vi "niRFSysCalReader Optimized Interpolation Method.vi"(0 "Max Delta Frequency, Hz":dbl=inf step=1000000.0 format="%^.6e", 1 "Max Delta Power Level, dBm":dbl=inf step=10.0 format="%.1f", 2 "Table (frequency, power, pathloss)":dbl[][](array[numeric]) caption="Calibration Table [Hz, dBm, dB]" min=0.0 max=127.0 format="%.2p", 3 "Max Input Power, dBm":dbl format="%.1f", 4 "Center Frequency, Hz":dbl=1000000000.0 step=1000000.0 format="%^.6e") -> (5 "Max Frequency Delta Reached?":bool, 6 "Max Power Delta Reached?":bool, 7 "External Attenuation, dB":dbl format="%.2f")   [LabVIEW 2016, in "niRFSysCalReader.lvlib"]
uses:
  niRFSysCalReader.lvlib
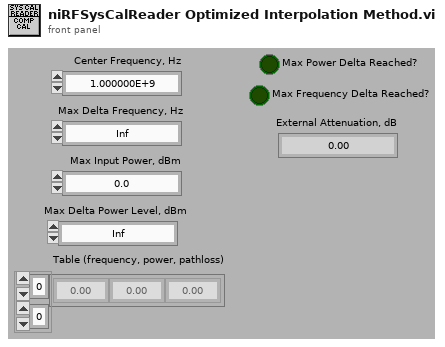
[diagram p1: front panel]
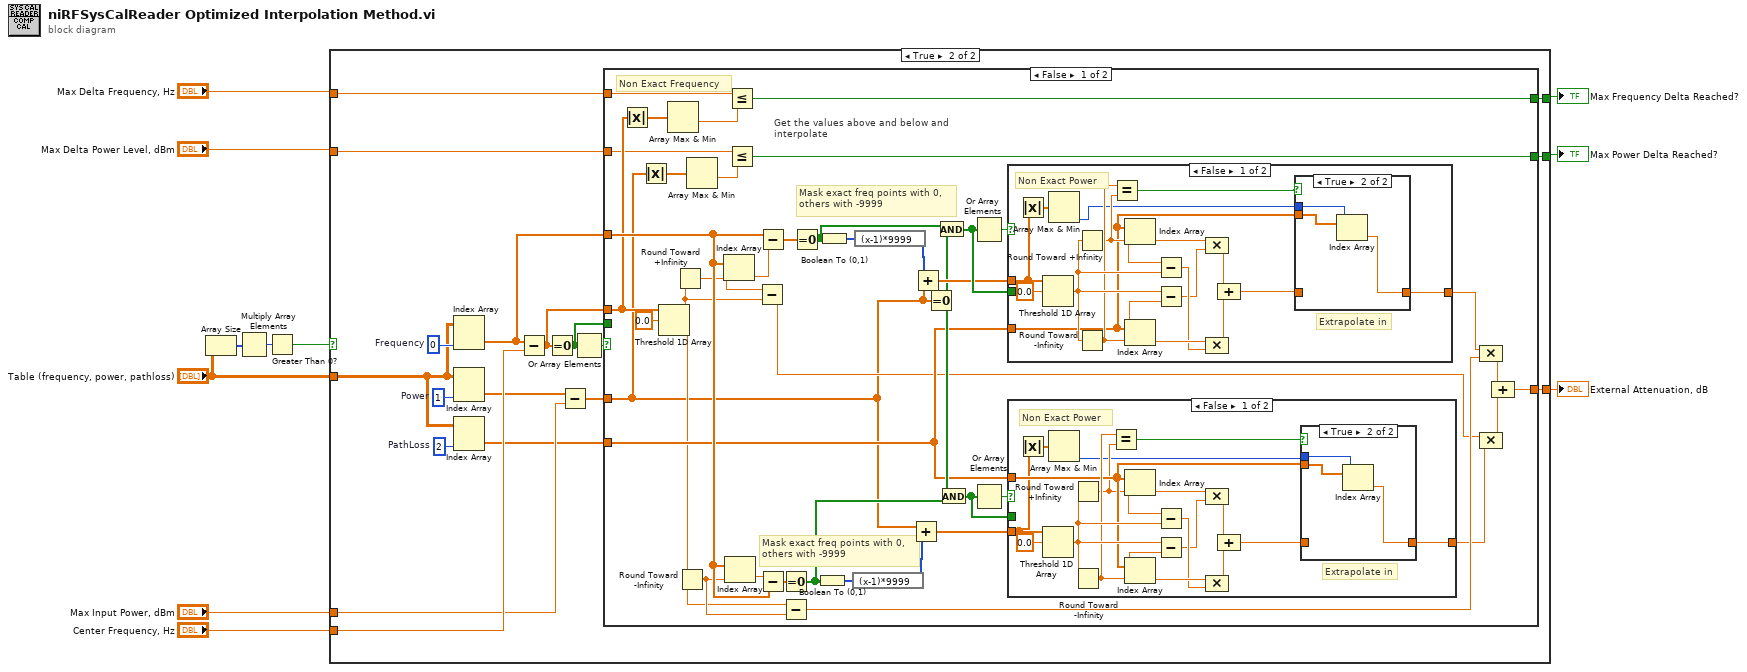
[diagram p0: block diagram]
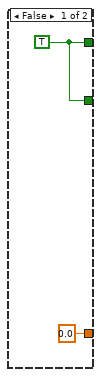
[diagram p2: hidden frame]
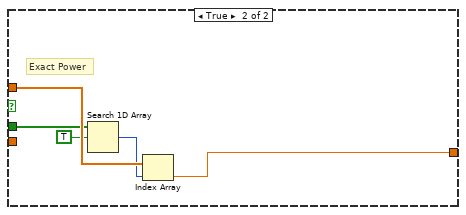
[diagram p4: hidden frame]
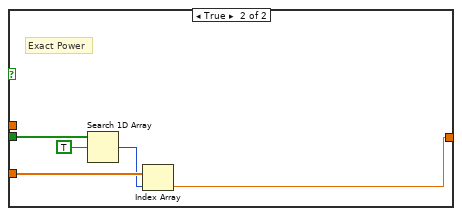
[diagram p6: hidden frame]
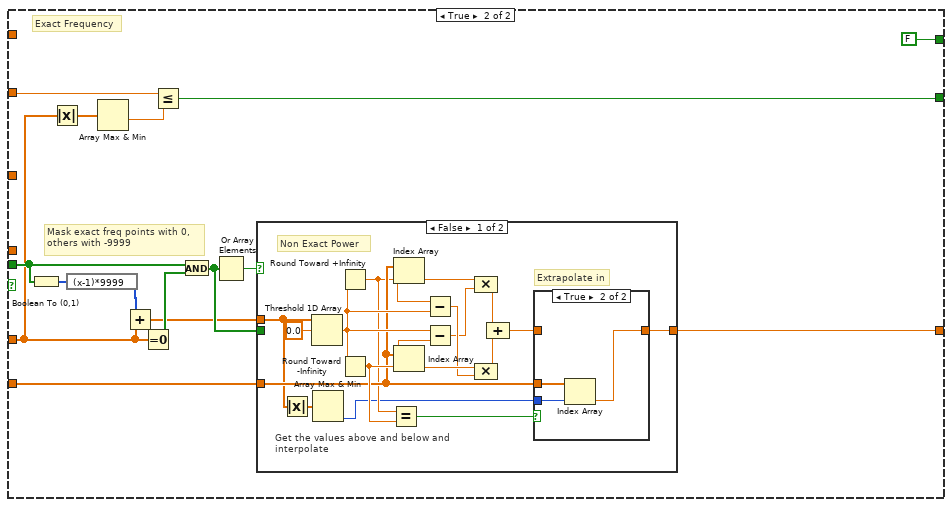
[diagram p7: hidden frame]
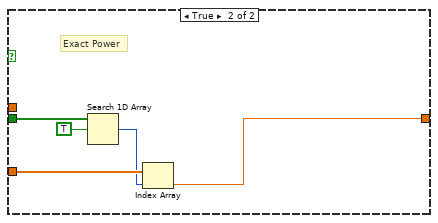
[diagram p9: hidden frame]
diagram:
  n1 = Array Size(array="Table (frequency, power, pathloss)") -> (size(s)=w3:i32[])
  n2 = Multiply Array Elements(1:w3) -> (0:w2:i32)
  n3 = Greater Than 0?(x=w2) -> (x > 0?=w1:bool)
  n4 = case shown="True" w1 {
    tunnel: [w13 w31] -> w11
    tunnel: [w13 w30] -> w10
    tunnel: "Center Frequency, Hz" -> [_ w29]
    tunnel: "Max Delta Power Level, dBm" -> [_ w28]
    tunnel: "Max Delta Frequency, Hz" -> [_ w27]
    tunnel: "Max Input Power, dBm" -> [_ w25]
    tunnel: [0.0 w23] -> w5
    tunnel: "Table (frequency, power, pathloss)" -> [_ w14]
    frame False {
      w13 = TRUE
    }
    frame True {
      w16 = 2  # PathLoss
      w15 = 0  # Frequency
      w17 = 1  # Power
      n5 = Index Array(array=w14, index (col)=w15) -> (element=w21:dbl[])  [unwired: 1 in]
      n6 = Index Array(array=w14, index (col)=w17) -> (element=w24:dbl[])  [unwired: 1 in]
      n7 = Index Array(array=w14, index (col)=w16) -> (element=w22:dbl[])  [unwired: 1 in]
      n8 = Subtract(x=w21, y=w29) -> (x-y=w20:dbl[])
      n9 = Equal To 0?(x=w20) -> (x = 0?=w19:bool[])
      n10 = Subtract(x=w24, y=w25) -> (x-y=w26:dbl[])
      n11 = Or Array Elements(Boolean array=w19) -> (logical OR=w18:bool)
      n12 = case shown="False" w18 {
        tunnel: w20 -> [w40 _]
        tunnel: w19 -> [_ w134]
        tunnel: w21 -> [w59 _]
        tunnel: w26 -> [w35 w126]
        tunnel: w22 -> [w53 w138]
        tunnel: [w43 w137] -> w23
        tunnel: w27 -> [w41 _]
        tunnel: w28 -> [w34 w127]
        tunnel: [w38 FALSE] -> w30
        tunnel: [w32 w125] -> w31
        frame False {
          # "Mask exact freq points with 0,\nothers with -9999"
          # "Mask exact freq points with 0,\nothers with -9999"
          # "Get the values above and below and\ninterpolate"
          # "Non Exact Frequency"
          n13 = Absolute Value(x=w40) -> (abs(x)=w39:dbl[])
          n14 = Absolute Value(x=w35) -> (abs(x)=w36:dbl[])
          n15 = Threshold 1D Array(2:0.0 ("threshold y"), 3:w40) -> (0:w44:dbl)  [unwired: 1 out]
          n16 = Array Max & Min(array=w39) -> (min value=w37:dbl)  [unwired: 3 out]
          n17 = Round Toward +Infinity(x=w44) -> (ceil(x): smallest int >= x=w45:dbl)
          n18 = Round Toward -Infinity(1:w44) -> (0:w46:dbl)
          n19 = Array Max & Min(array=w36) -> (min value=w33:dbl)  [unwired: 3 out]
          n20 = Index Array(array=w59, index=w45) -> (element=w42:dbl)
          n21 = Index Array(array=w59, index=w46) -> (element=w60:dbl)
          n22 = Less Or Equal?(x=w41, y=w37) -> (x <= y?=w38:bool)
          n23 = Less Or Equal?(x=w34, y=w33) -> (x <= y?=w32:bool)
          n24 = Subtract(x=w45, y=w44) -> (x-y=w47:dbl)
          n25 = Subtract(x=w59, y=w42) -> (x-y=w65:dbl[])
          n26 = Subtract(x=w60, y=w59) -> (x-y=w63:dbl[])
          n27 = Equal To 0?(x=w63) -> (x = 0?=w57:bool[])
          n28 = Subtract(x=w44, y=w46) -> (x-y=w52:dbl)
          n29 = Equal To 0?(x=w65) -> (x = 0?=w64:bool[])
          n30 = Boolean To (0,1)(Boolean=w57) -> (0, 1=w61:i16[])
          n31 = Boolean To (0,1)(Boolean=w64) -> (0, 1=w68:i16[])
          n32 = expression code="(x-1)*9999"(w61) -> (w62:i16[])
          n33 = expression code="(x-1)*9999"(w68) -> (w67:i16[])
          n34 = Add(x=w35, y=w62) -> (x+y=w54:dbl[])
          n35 = Add(x=w67, y=w35) -> (x+y=w66:dbl[])
          n36 = Equal To 0?(x=w35) -> (x = 0?=w58:bool[])
          n37 = And(x=w64, y=w58) -> (x .and. y?=w69:bool[])
          n38 = And(x=w58, y=w57) -> (x .and. y?=w55:bool[])
          n39 = Or Array Elements(Boolean array=w69) -> (logical OR=w70:bool)
          n40 = Or Array Elements(Boolean array=w55) -> (logical OR=w56:bool)
          n41 = case shown="False" w70 {
            tunnel: w53 -> [w103 w123]
            tunnel: [w101 w122] -> w49
            tunnel: w69 -> [_ w121]
            tunnel: w66 -> [w99 _]
            frame False {
              # "Extrapolate in"
              # "Non Exact Power"
              n42 = Absolute Value(x=w99) -> (abs(x)=w100:dbl[])
              n43 = Threshold 1D Array(2:0.0 ("threshold y"), 3:w99) -> (0:w111:dbl)  [unwired: 1 out]
              n44 = Array Max & Min(array=w100) -> (min index (indices)=w98:i32)  [unwired: 3 out]
              n45 = Round Toward +Infinity(x=w111) -> (ceil(x): smallest int >= x=w104:dbl)
              n46 = Round Toward -Infinity(1:w111) -> (0:w106:dbl)
              n47 = Equal?(x=w106, y=w104) -> (x = y?=w105:bool)
              n48 = Index Array(array=w103, index=w104) -> (element=w113:dbl)
              n49 = Index Array(array=w103, index=w106) -> (element=w112:dbl)
              n50 = Subtract(x=w104, y=w111) -> (x-y=w108:dbl)
              n51 = Subtract(x=w111, y=w106) -> (x-y=w107:dbl)
              n52 = Compound Arithmetic op=MULTIPLY(w113, w107) -> (w110:dbl)
              n53 = Compound Arithmetic op=MULTIPLY(w112, w108) -> (w109:dbl)
              n54 = Compound Arithmetic op=ADD(w110, w109) -> (w102:dbl)
              n55 = case shown="True" w105 {
                tunnel: w102 -> [w115 _]
                tunnel: [w115 w118] -> w101
                tunnel: w98 -> [_ w116]
                tunnel: w103 -> [_ w117]
                frame False {
                }
                frame True {
                  n56 = Index Array(array=w117, index=w116) -> (element=w118:dbl)
                }
              }
            }
            frame True {
              # "Exact Power"
              n57 = Search 1D Array(1D array=w121, element=TRUE) -> (index of element=w119:i32)  [unwired: 1 out]
              n58 = Index Array(array=w123, index=w119) -> (element=w122:dbl)
            }
          }
          n59 = case shown="False" w56 {
            tunnel: w53 -> [w76 w97]
            tunnel: [w79 w96] -> w48
            tunnel: w55 -> [_ w95]
            tunnel: w54 -> [w74 _]
            frame False {
              # "Extrapolate in"
              # "Non Exact Power"
              n60 = Absolute Value(x=w74) -> (abs(x)=w75:dbl[])
              n61 = Threshold 1D Array(2:0.0 ("threshold y"), 3:w74) -> (0:w85:dbl)  [unwired: 1 out]
              n62 = Array Max & Min(array=w75) -> (min index (indices)=w72:i32)  [unwired: 3 out]
              n63 = Round Toward +Infinity(x=w85) -> (ceil(x): smallest int >= x=w73:dbl)
              n64 = Round Toward -Infinity(1:w85) -> (0:w78:dbl)
              n65 = Equal?(x=w78, y=w73) -> (x = y?=w77:bool)
              n66 = Index Array(array=w76, index=w73) -> (element=w87:dbl)
              n67 = Index Array(array=w76, index=w78) -> (element=w86:dbl)
              n68 = Subtract(x=w73, y=w85) -> (x-y=w82:dbl)
              n69 = Subtract(x=w85, y=w78) -> (x-y=w81:dbl)
              n70 = Compound Arithmetic op=MULTIPLY(w87, w81) -> (w84:dbl)
              n71 = Compound Arithmetic op=MULTIPLY(w86, w82) -> (w83:dbl)
              n72 = Compound Arithmetic op=ADD(w84, w83) -> (w80:dbl)
              n73 = case shown="True" w77 {
                tunnel: w80 -> [w89 _]
                tunnel: [w89 w92] -> w79
                tunnel: w72 -> [_ w90]
                tunnel: w76 -> [_ w91]
                frame False {
                }
                frame True {
                  n74 = Index Array(array=w91, index=w90) -> (element=w92:dbl)
                }
              }
            }
            frame True {
              # "Exact Power"
              n75 = Search 1D Array(1D array=w95, element=TRUE) -> (index of element=w93:i32)  [unwired: 1 out]
              n76 = Index Array(array=w97, index=w93) -> (element=w96:dbl)
            }
          }
          n77 = Compound Arithmetic op=MULTIPLY(w49, w52) -> (w50:dbl)
          n78 = Compound Arithmetic op=MULTIPLY(w47, w48) -> (w51:dbl)
          n79 = Compound Arithmetic op=ADD(w50, w51) -> (w43:dbl)
        }
        frame True {
          # "Mask exact freq points with 0,\nothers with -9999"
          # "Exact Frequency"
          n80 = Boolean To (0,1)(Boolean=w134) -> (0, 1=w132:i16[])
          n81 = Absolute Value(x=w126) -> (abs(x)=w129:dbl[])
          n82 = expression code="(x-1)*9999"(w132) -> (w131:i16[])
          n83 = Array Max & Min(array=w129) -> (min value=w128:dbl)  [unwired: 3 out]
          n84 = Add(x=w131, y=w126) -> (x+y=w130:dbl[])
          n85 = Equal To 0?(x=w126) -> (x = 0?=w133:bool[])
          n86 = Less Or Equal?(x=w127, y=w128) -> (x <= y?=w125:bool)
          n87 = And(x=w134, y=w133) -> (x .and. y?=w135:bool[])
          n88 = Or Array Elements(Boolean array=w135) -> (logical OR=w136:bool)
          n89 = case shown="False" w136 {
            tunnel: w138 -> [w144 w164]
            tunnel: [w142 w163] -> w137
            tunnel: w135 -> [_ w162]
            tunnel: w130 -> [w141 _]
            frame False {
              # "Extrapolate in"
              # "Get the values above and below and\ninterpolate"
              # "Non Exact Power"
              n90 = Absolute Value(x=w141) -> (abs(x)=w140:dbl[])
              n91 = Threshold 1D Array(2:0.0 ("threshold y"), 3:w141) -> (0:w152:dbl)  [unwired: 1 out]
              n92 = Array Max & Min(array=w140) -> (min index (indices)=w139:i32)  [unwired: 3 out]
              n93 = Round Toward +Infinity(x=w152) -> (ceil(x): smallest int >= x=w143:dbl)
              n94 = Round Toward -Infinity(1:w152) -> (0:w147:dbl)
              n95 = Equal?(x=w143, y=w147) -> (x = y?=w146:bool)
              n96 = Index Array(array=w144, index=w143) -> (element=w154:dbl)
              n97 = Index Array(array=w144, index=w147) -> (element=w153:dbl)
              n98 = Subtract(x=w143, y=w152) -> (x-y=w149:dbl)
              n99 = Subtract(x=w152, y=w147) -> (x-y=w148:dbl)
              n100 = Compound Arithmetic op=MULTIPLY(w154, w148) -> (w151:dbl)
              n101 = Compound Arithmetic op=MULTIPLY(w153, w149) -> (w150:dbl)
              n102 = Compound Arithmetic op=ADD(w151, w150) -> (w145:dbl)
              n103 = case shown="True" w146 {
                tunnel: w145 -> [w156 _]
                tunnel: w144 -> [_ w159]
                tunnel: w139 -> [_ w158]
                tunnel: [w156 w157] -> w142
                frame False {
                }
                frame True {
                  n104 = Index Array(array=w159, index=w158) -> (element=w157:dbl)
                }
              }
            }
            frame True {
              # "Exact Power"
              n105 = Search 1D Array(1D array=w162, element=TRUE) -> (index of element=w160:i32)  [unwired: 1 out]
              n106 = Index Array(array=w164, index=w160) -> (element=w163:dbl)
            }
          }
        }
      }
    }
  }
  "Max Power Delta Reached?" <- w11
  "Max Frequency Delta Reached?" <- w10
  "External Attenuation, dB" <- w5
